vi "Init Hardware.vi"(8 "error in (no error)":errorcluster, 11 "Magnet Driver in":refnum<class "Magnet Driver.lvclass">) -> (0 "error out":errorcluster, 3 "Magnet Driver out":refnum<class "Magnet Driver.lvclass">)   [LabVIEW 2021, in "Magnet Driver.lvclass"]
uses:
  Magnet Driver.lvclass
  opt/github/NHMFL_Core/Libraries/Instruments/Instrument Driver/Instrument Driver.lvclass
  Instrument Driver/Instrument Driver.lvclass/Instrument Driver.ctl
  Instrument Driver/Read Recorder name.vi
  Instrument Driver/Write Channel names.vi
  Instrument Driver/Write Channel units.vi
  Simple VISA Reader/Simple VISA Reader Driver.lvclass
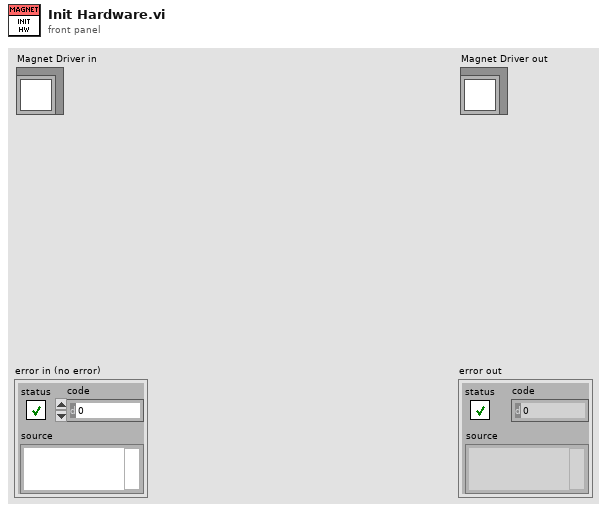
[diagram p1: front panel]
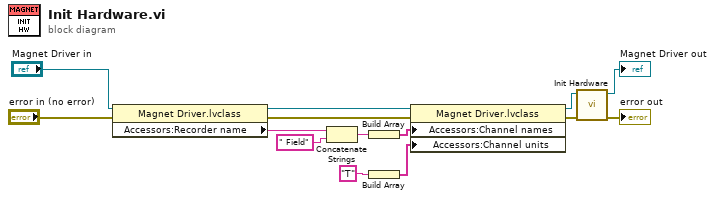
[diagram p0: block diagram]
diagram:
  n1 = property class="Magnet Driver.lvclass"(reference="Magnet Driver in", error in="error in (no error)") -> (reference out=w9:refnum<class "Magnet Driver.lvclass">, error out=w10:errorcluster, "Accessors:Recorder name"=w12:string)
  n2 = Concatenate Strings(w12, " Field") -> (w11:string)
  n3 = Build Array(w11) -> (w6:string[])
  n4 = Build Array("T") -> (w8:string[])
  n5 = property class="Magnet Driver.lvclass"(reference=w9, error in=w10, "Accessors:Channel names"=w6, "Accessors:Channel units"=w8) -> (reference out=w4:refnum<class "Magnet Driver.lvclass">, error out=w1:errorcluster)
  n6 = call-parent "Init Hardware.vi"("error in (no error)"=w1, "Instrument Driver in"=w4) -> ("error out"=→"error out":errorcluster, "Instrument Driver out"=→"Magnet Driver out":refnum<class "Magnet Driver.lvclass">)  [unwired: 8 in]
